vi "Untitled 3.vi"() -> ()   [LabVIEW 2021]
panel:
  out "substring 2":string
  out "USER STRING":string
  out "TIME":sgl format="%<%H:%M:%S>t"
  out "value":sgl[](array[numeric]) format="%#_6f"
  out "LATITUDE":sgl
  out "LONGITUTED":sgl
  out "value 2":i8
  out "value 3":i16
  out "HEADING":sgl
  out "substring":string
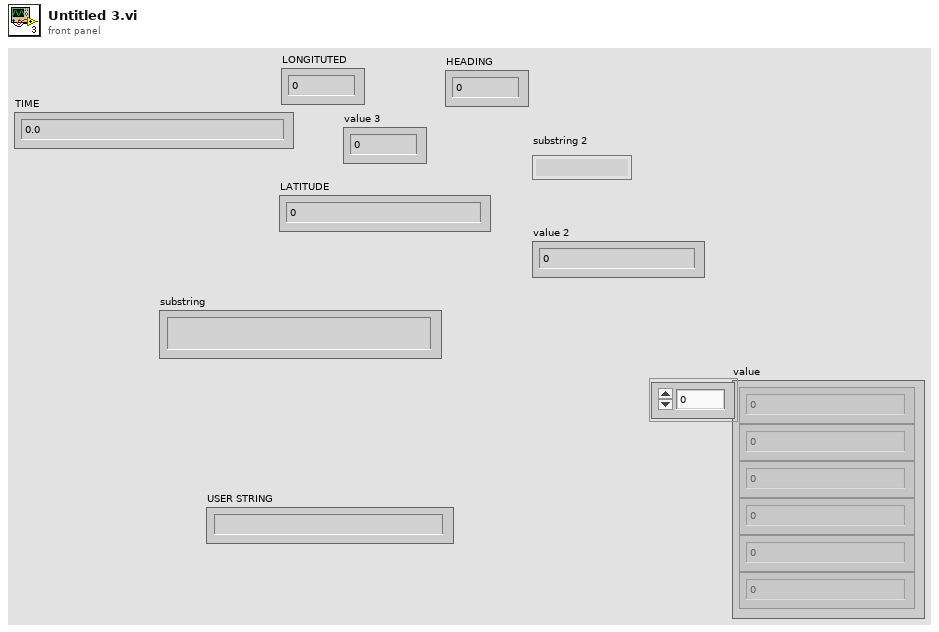
[diagram p1: front panel]
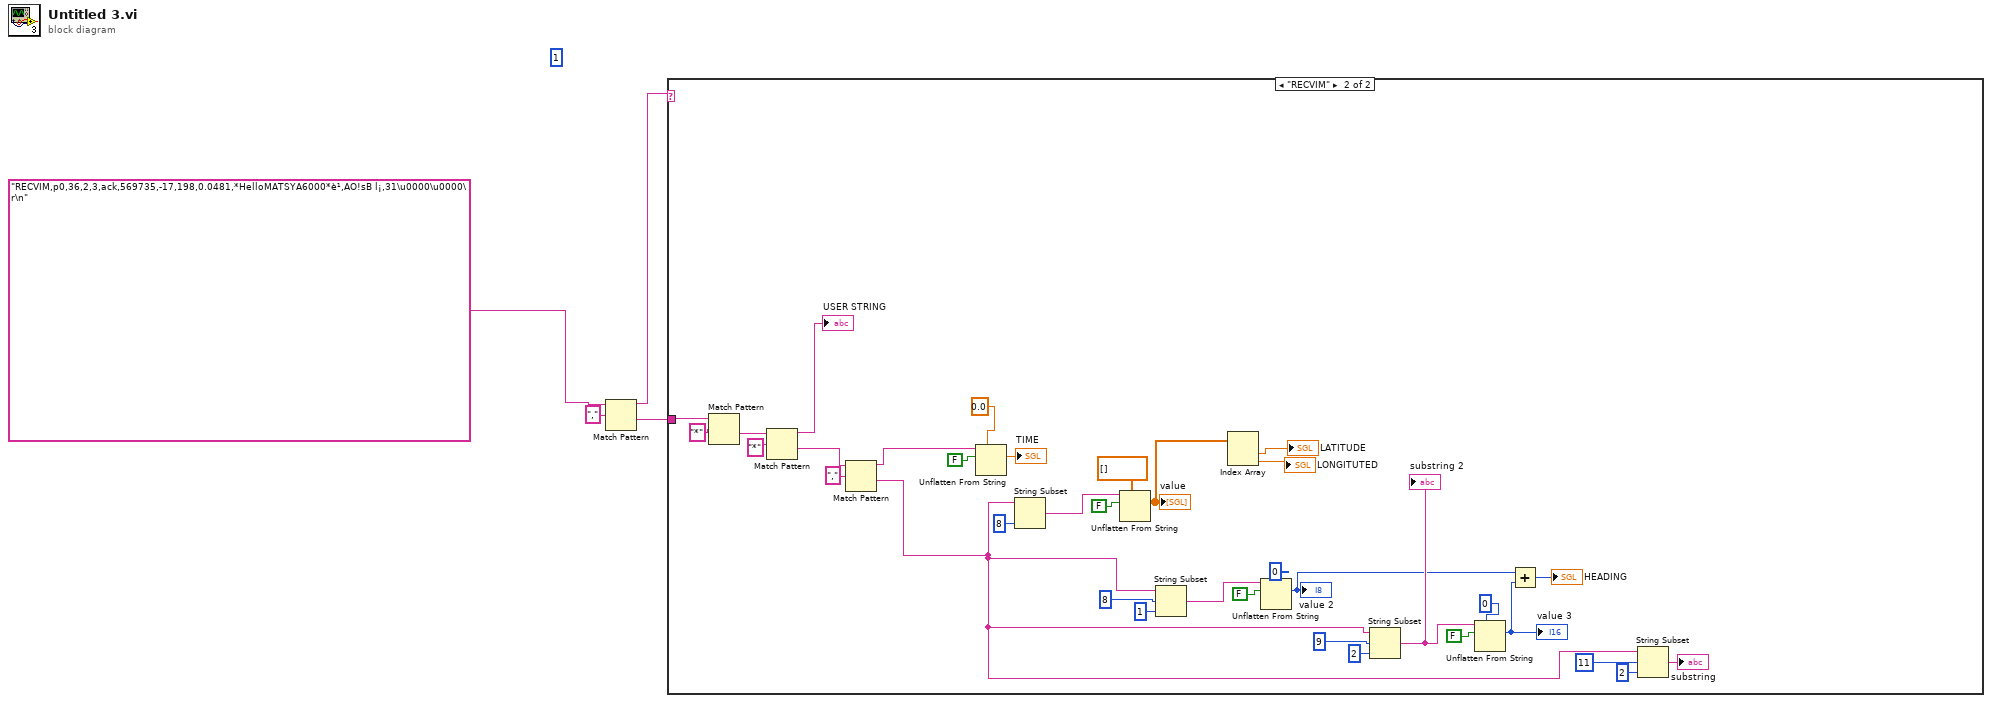
[diagram p0: block diagram]
diagram:
  (unwired) 1
  n1 = Match Pattern(string="RECVIM,p0,36,2,3,ack,569735,-17,198,0.0481,*HelloMATSYA6000*è¹,AO!sB l¡,31\u0000\u0000\r\n", regular expression=",") -> (before substring=w2:string, after substring=w1:string)  [unwired: 1 in, 2 out]
  n2 = case shown="\"RECVIM\"" w2 {
    tunnel: w1 -> [_ w39]
    frame "USBLANGLES", Default {
    }
    frame "RECVIM" {
      n3 = Match Pattern(string=w39, regular expression="*") -> (after substring=w36:string)  [unwired: 1 in, 3 out]
      n4 = Match Pattern(string=w36, regular expression="*") -> (before substring=→"USER STRING":string, after substring=w7:string)  [unwired: 1 in, 2 out]
      n5 = Match Pattern(string=w7, regular expression=",") -> (before substring=w6:string, after substring=w5:string)  [unwired: 1 in, 2 out]
      n6 = Unflatten From String(type=sgl 0.0, binary string=w6, data includes array or string size? (T)=FALSE) -> (value=→"TIME":sgl)  [unwired: 2 in, 2 out]
      n7 = String Subset(string=w5, length (rest)=8 ("length (rest)")) -> (substring=w29:string)  [unwired: 1 in]
      n8 = Unflatten From String(type=sgl[] [], binary string=w29, data includes array or string size? (T)=FALSE) -> (value=w27:sgl[])  [unwired: 2 in, 2 out]
      "value" <- w27
      n9 = String Subset(string=w5, offset (0)=8 ("length (rest)"), length (rest)=1 ("length (rest)")) -> (substring=w23:string)
      n10 = Index Array(array=w27) -> (element #1=→"LATITUDE":sgl, element #2=→"LONGITUTED":sgl)  [unwired: 2 in]
      n11 = Unflatten From String(type=i8 0, binary string=w23, data includes array or string size? (T)=FALSE) -> (value=w14:i8)  [unwired: 2 in, 2 out]
      "value 2" <- w14
      n12 = String Subset(string=w5, offset (0)=9 ("length (rest)"), length (rest)=2 ("length (rest)")) -> (substring=w18:string)
      "substring 2" <- w18
      n13 = Unflatten From String(type=i16 0, binary string=w18, data includes array or string size? (T)=FALSE) -> (value=w15:i16)  [unwired: 2 in, 2 out]
      "value 3" <- w15
      n14 = Add(x=w14, y=w15) -> (x+y=→"HEADING":i16)
      n15 = String Subset(string=w5, offset (0)=11 ("length (rest)"), length (rest)=2 ("length (rest)")) -> (substring=→"substring":string)
    }
  }
